vi "test Write and Read Unsigned Integer.vi"(8 "error in (no error)":errorcluster, 11 "TestCase in":refnum<class "Read Value Tests.lvclass">) -> (0 "error out":errorcluster, 3 "TestCase out":refnum<class "Read Value Tests.lvclass">)   [LabVIEW 2020, in "Memory Manager Tests.lvlib" / "Read Value Tests.lvclass"]
uses:
  Read Value Tests.lvclass
  Read Value Tests.lvclass/Read Value Tests.ctl
  C:/Program Files/National Instruments/LabVIEW 2027/vi.lib/addons/_JKI Toolkits/VI Tester/TestCase.llb/TestCase.lvclass
  <vilib>/addons/_JKI Toolkits/VI Tester/TestCase.llb/TestCase.lvclass
  Classes/Pointer/Pointer.lvclass
  Classes/Pointer/Read U8.vi
  Classes/Pointer/Read U16.vi
  Classes/Pointer/Read U32.vi
  Classes/Pointer/Read U64.vi
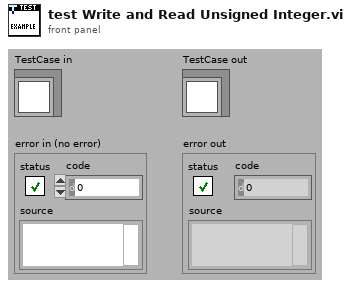
[diagram p1: front panel]
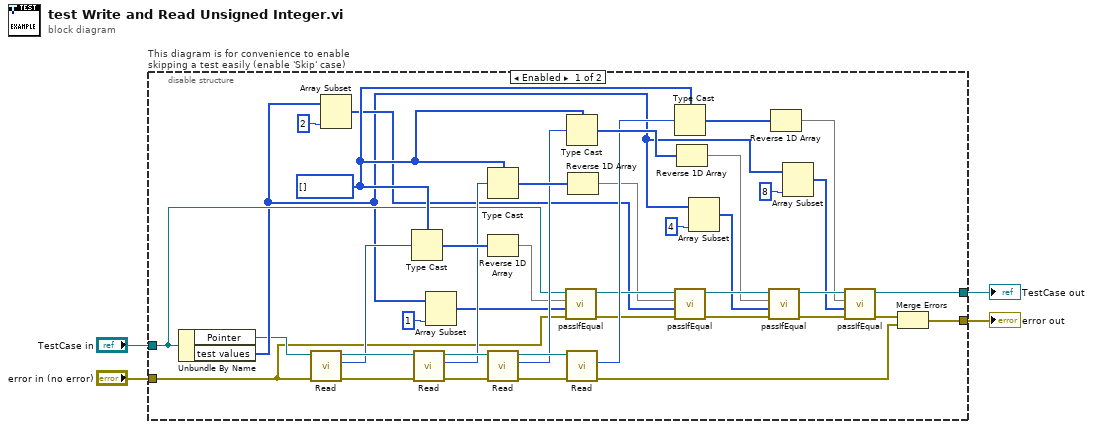
[diagram p0: block diagram]
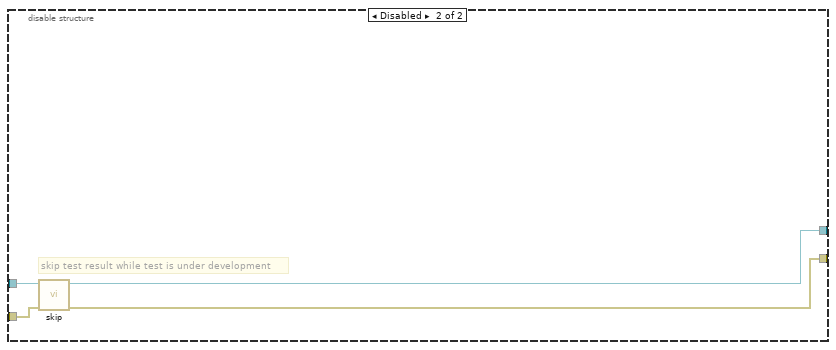
[diagram p2: hidden frame]
diagram:
  n1 = disable-structure "This diagram is for convenience to enable skipping a test easily (enable 'Skip' case)" shown="Enabled" {
    disable-tunnel: "TestCase in" -> [w10 w49]
    disable-tunnel: [w11 w47] -> w1
    disable-tunnel: [w6 w48] -> w3
    disable-tunnel: "error in (no error)" -> [w7 w46]
    frame Enabled {
      w28 = u8[] [] ("buffer in")
      n2 = Unbundle By Name(w10) -> ("Pointer"=w8:refnum<class "Pointer.lvclass">, "test values"=w9:u8[])
      n3 = call-poly "Read.vi"("error in (no error)"=w7, "Pointer in"=w8) -> ("error out"=w41:errorcluster, "value out"=w32:u8, "Pointer out"=w42:refnum<class "Pointer.lvclass">)  [unwired: 6 in, 1 out]
      n4 = Array Subset(array=w9, length=2) -> (w17:u8[])  [unwired: 1 in]
      n5 = Type Cast(type=w28, x=w32) -> (*(type *) &x=w36:u8[])
      n6 = call-poly "Read.vi"("error in (no error)"=w41, "Pointer in"=w42) -> ("error out"=w39:errorcluster, "value out"=w31:u16, "Pointer out"=w40:refnum<class "Pointer.lvclass">)  [unwired: 6 in, 1 out]
      n7 = Array Subset(array=w9, length=1) -> (w18:u8[])  [unwired: 1 in]
      n8 = Type Cast(type=w28, x=w31) -> (*(type *) &x=w35:u8[])
      n9 = Reverse 1D Array(array=w36) -> (reversed array=w20:u8[])
      n10 = call-poly "Read.vi"("error in (no error)"=w39, "Pointer in"=w40) -> ("error out"=w37:errorcluster, "value out"=w30:u32, "Pointer out"=w38:refnum<class "Pointer.lvclass">)  [unwired: 6 in, 1 out]
      n11 = call-dynamic "passIfEqual.vi"("error in (no error)"=w7, "y"=w18, "x"=w20, "TestCase in"=w10) -> ("error out"=w23:errorcluster, "TestCase out"=w24:refnum<class "Read Value Tests.lvclass">)  [unwired: 6 in]
      n12 = Type Cast(type=w28, x=w30) -> (*(type *) &x=w34:u8[])
      n13 = call-poly "Read.vi"("error in (no error)"=w37, "Pointer in"=w38) -> ("error out"=w5:errorcluster, "value out"=w29:u64)  [unwired: 6 in, 2 out]
      n14 = Reverse 1D Array(array=w35) -> (reversed array=w19:u8[])
      n15 = Type Cast(type=w28, x=w29) -> (*(type *) &x=w33:u8[])
      n16 = call-dynamic "passIfEqual.vi"("error in (no error)"=w23, "y"=w17, "x"=w19, "TestCase in"=w24) -> ("error out"=w21:errorcluster, "TestCase out"=w22:refnum<class "Read Value Tests.lvclass">)  [unwired: 6 in]
      n17 = Reverse 1D Array(array=w34) -> (reversed array=w15:u8[])
      n18 = Array Subset(array=w9, length=4) -> (w16:u8[])  [unwired: 1 in]
      n19 = call-dynamic "passIfEqual.vi"("error in (no error)"=w21, "y"=w16, "x"=w15, "TestCase in"=w22) -> ("error out"=w26:errorcluster, "TestCase out"=w25:refnum<class "Read Value Tests.lvclass">)  [unwired: 6 in]
      n20 = Reverse 1D Array(array=w33) -> (reversed array=w13:u8[])
      n21 = Array Subset(array=w9, length=8) -> (w14:u8[])  [unwired: 1 in]
      n22 = call-dynamic "passIfEqual.vi"("error in (no error)"=w26, "y"=w14, "x"=w13, "TestCase in"=w25) -> ("error out"=w12:errorcluster, "TestCase out"=w11:refnum<class "Read Value Tests.lvclass">)  [unwired: 6 in]
      n23 = Merge Errors(w12, w5) -> (w6:errorcluster)
    }
    frame Disabled {
      # "skip test result while test is under development"
      n24 = call <vilib>:"skip.vi"("error in (no error)"=w46, "TestCase in"=w49) -> ("error out"=w48:errorcluster, "TestCase out"=w47:refnum<class "Read Value Tests.lvclass">)  [unwired: 8 in]
    }
  }
  "error out" <- w3
  "TestCase out" <- w1
